vi "Johnson_lindenstrauss_min_dim.vi"(10 "Eps":sgl, 11 "N_Samples":i32) -> (3 "jl_min_Dim":i32)   [LabVIEW 2020]
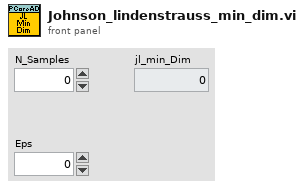
[diagram p1: front panel]
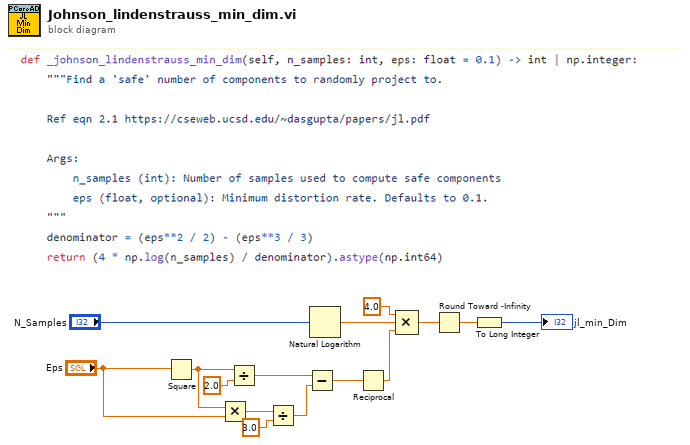
[diagram p0: block diagram]
diagram:
  n1 = Square(x="Eps") -> (x^2=w13:sgl)
  n2 = Multiply(x=w13, y="Eps") -> (x*y=w10:sgl)
  n3 = Divide(x=w13, y=sgl 2.0) -> (x/y=w14:sgl)
  n4 = Divide(x=w10, y=sgl 3.0) -> (x/y=w9:sgl)
  n5 = Subtract(x=w14, y=w9) -> (x-y=w8:sgl)
  n6 = Natural Logarithm(1:"N_Samples") -> (0:w5:dbl)
  n7 = Reciprocal(x=w8) -> (1/x=w6:sgl)
  n8 = Compound Arithmetic op=MULTIPLY(4.0 ("value"), w5, w6) -> (w2:dbl)
  n9 = Round Toward -Infinity(1:w2) -> (0:w1:dbl)
  n10 = To Long Integer(number=w1) -> (32bit integer=→"jl_min_Dim":i32)
